vi "Configure Measurement.vi"   [LabVIEW 2022 SP3, in "Agilent N934X Series.lvlib"]
doc: "This is a poly VI for configure measurement VIs."
uses:
  <instrlib>/Agilent N934X Series/Agilent N934X Series.lvlib
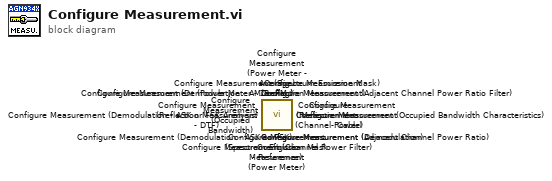
[diagram p0: block diagram]
diagram:
  n1 = call <instrlib>:"Configure Measurement (Spectrum Emission Mask - Reference).vi"() -> ()  [unwired: 14 in, 2 out]
  n2 = call <instrlib>:"Configure Measurement (Reflection Measurement).vi"() -> ()  [unwired: 14 in, 2 out]
  n3 = call <instrlib>:"Configure Measurement (Reflection Measurement - DTF).vi"() -> ()  [unwired: 14 in, 2 out]
  n4 = call <instrlib>:"Configure Measurement (Reflection Measurement - Cable).vi"() -> ()  [unwired: 14 in, 2 out]
  n5 = call <instrlib>:"Configure Measurement (Power Meter - Zeroing).vi"() -> ()  [unwired: 14 in, 2 out]
  n6 = call <instrlib>:"Configure Measurement (Power Meter - Average).vi"() -> ()  [unwired: 14 in, 2 out]
  n7 = call <instrlib>:"Configure Measurement (Demodulation).vi"() -> ()  [unwired: 14 in, 2 out]
  n8 = call <instrlib>:"Configure Measurement (Demodulation - ASK or FSK).vi"() -> ()  [unwired: 14 in, 2 out]
  n9 = call <instrlib>:"Configure Measurement (Demodulation - ASK or FSK Analysis).vi"() -> ()  [unwired: 14 in, 2 out]
  n10 = call <instrlib>:"Configure Measurement (Occupied Bandwidth Characteristics).vi"() -> ()  [unwired: 14 in, 2 out]
  n11 = call <instrlib>:"Configure Measurement (Channel Power Filter).vi"() -> ()  [unwired: 14 in, 2 out]
  n12 = call <instrlib>:"Configure Measurement (Adjacent Channel Power Ratio Filter).vi"() -> ()  [unwired: 14 in, 2 out]
  n13 = call <instrlib>:"Configure Measurement (Spectrum Emission Mask).vi"() -> ()  [unwired: 14 in, 2 out]
  n14 = call <instrlib>:"Configure Measurement (Power Meter).vi"() -> ()  [unwired: 14 in, 2 out]
  n15 = call <instrlib>:"Configure Measurement (Demodulation - AM or FM ).vi"() -> ()  [unwired: 14 in, 2 out]
  n16 = call <instrlib>:"Configure Measurement (Adjacent Channel Power Ratio).vi"() -> ()  [unwired: 14 in, 2 out]
  n17 = call <instrlib>:"Configure Measurement (Occupied Bandwidth).vi"() -> ()  [unwired: 14 in, 2 out]
  n18 = call <instrlib>:"Configure Measurement (Channel Power).vi"() -> ()  [unwired: 14 in, 2 out]
